vi "initialize_console.vi"(8 "error in (no error)":errorcluster, 11 "console (in)":refnum<vi>) -> (0 "error out":errorcluster, 3 "reference out":refnum<vi>)   [LabVIEW 2021, in "console.provider.lvclass"]
uses:
  console.provider.lvclass
  console.provider.lvclass/console.provider.ctl
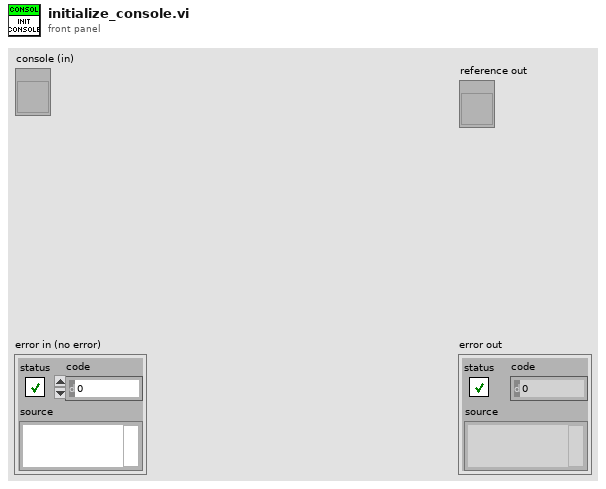
[diagram p1: front panel]
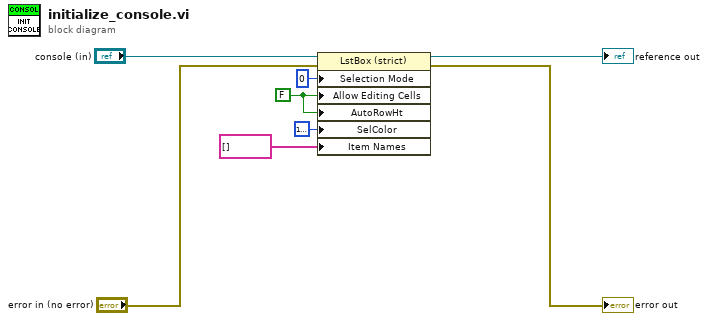
[diagram p0: block diagram]
diagram:
  w3 = FALSE ("Allow Editing Cells")
  n1 = property class="LstBox (strict)"(reference="console (in)", error in="error in (no error)", "Selection Mode"=0, "Allow Editing Cells"=w3, "AutoRowHt"=w3, "SelColor"=u32 16777216 ("Selection Color"), "Item Names"=string[] []) -> (reference out=→"reference out":refnum<vi>, error out=→"error out":errorcluster)
